vi "lopp execution time check.vi"(8 "?":T1=enum."PLC_com") -> (0 "?":T1[](array[typedef]), 1 "appended array":u32[](array[numeric]))   [LabVIEW 2017]
uses:
  Controls/Station_wise_live_breakdown_loop.ctl
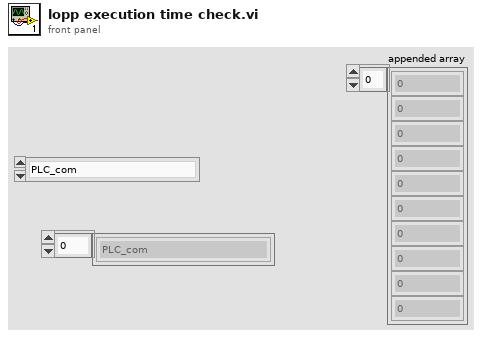
[diagram p1: front panel]
types:
  T1 = typedef "Station_wise_live_breakdown_loop.ctl" = enum16{"Int_3", "Break_down", "Rejection_count", "STOP", "BUTTON_SWITCH", "Init_2", "Alaram_stat", "Product_count", "PLC_com", "Init", "Oven_Reading"}
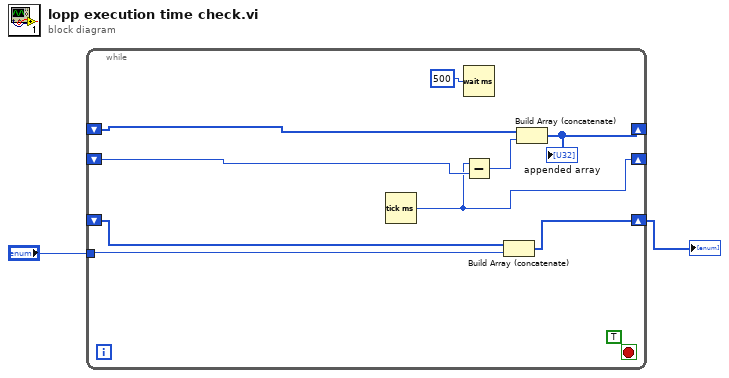
[diagram p0: block diagram]
diagram:
  n1 = while {
    shift-right: [w11] -> _
    shift-left: _ -> [w10]
    shift-right: [w7] -> _
    shift-left: _ -> [w8]
    tunnel: "?" -> [w4]
    shift-right: [w3] -> w1
    shift-left: _ -> [w5]
    stop <- TRUE ("stop") stop-if-true
    n2 = Tick Count (ms)() -> (millisecond timer value=w7:u32)
    n3 = Wait (ms)(milliseconds to wait=u32 500) -> ()  [unwired: 1 out]
    n4 = Subtract(x=w7, y=w8) -> (x-y=w6:u32)
    n5 = Build Array (concatenate)(w5, w4) -> (w3:T1[])
    n6 = Build Array (concatenate)(w10, w6) -> (w11:u32[])
    "appended array" <- w11
  }
  "?" <- w1
